vi "Set BasePath and AppName.vi"(8 "error in (no error)":errorcluster, 9 "ErrorLogBasePath":path, 10 "AppName":string, 11 "ErrorHandler in":refnum<class "ErrorHandler.lvclass">) -> (0 "error out":errorcluster, 3 "ErrorHandler out":refnum<class "ErrorHandler.lvclass">)   [LabVIEW 2019, in "ErrorHandler.lvclass"]
doc: "Developed by Kevin Thompson\nkevin@thompsonengineering.net\n\nCopyright 2018\nThompson Engineering, LLC"
uses:
  ErrorHandler.lvclass
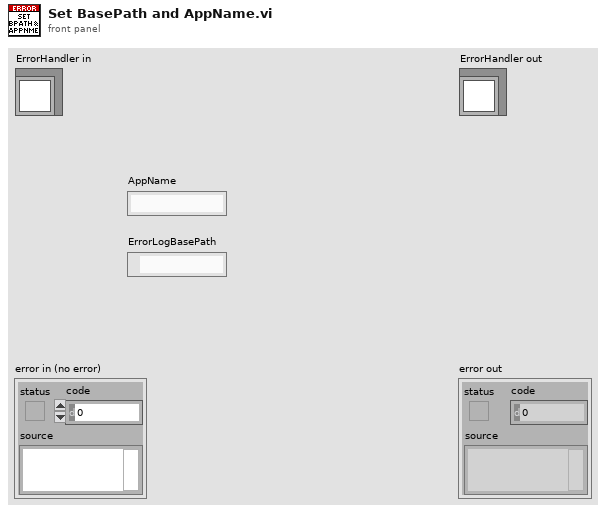
[diagram p1: front panel]
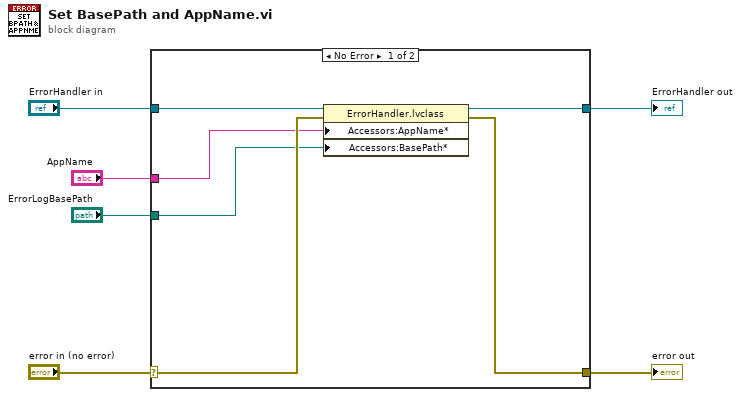
[diagram p0: block diagram]
diagram:
  n1 = case shown="No Error" "error in (no error)" {
    selector: "error in (no error)" -> [w10 w14]
    tunnel: [w9 w14] -> w5
    tunnel: [w11 w13] -> w3
    tunnel: "ErrorHandler in" -> [w12 w13]
    tunnel: "AppName" -> [w8 _]
    tunnel: "ErrorLogBasePath" -> [w7 _]
    frame No Error {
      n2 = property class="ErrorHandler.lvclass"(reference=w12, error in=w10, "Accessors:AppName*"=w8, "Accessors:BasePath*"=w7) -> (reference out=w11:refnum<class "ErrorHandler.lvclass">, error out=w9:errorcluster)
    }
    frame Error {
    }
  }
  "error out" <- w5
  "ErrorHandler out" <- w3
